vi "System_Read Module DVRs.vi"(11 "Data Value Reference in":refnum<data-value>) -> (2 "Dispatch Module DVR Array":refnum<data-value>[](array[refnum]), 3 "Data Value Reference out":refnum<data-value>)   [LabVIEW 2015, in "System.lvclass"]
uses:
  System.lvclass
  DispatchInterface/Interface_Dispatch.lvclass
  System.lvclass/System.ctl
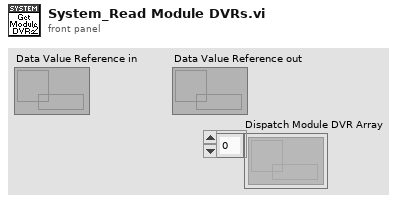
[diagram p1: front panel]
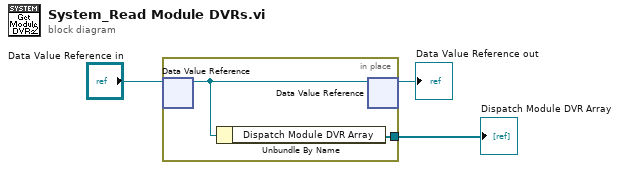
[diagram p0: block diagram]
diagram:
  n1 = in-place {
    in-place-border: [w4] -> w1
    n2 = in-place-dvr #1("Data Value Reference in") -> (w5:refnum<class "System.lvclass">)  [unwired: 1 out]
    n3 = Unbundle By Name(w5) -> ("Dispatch Module DVR Array"=w4:refnum<data-value>[])
    n4 = in-place-dvr #1(w5) -> (→"Data Value Reference out":refnum<data-value>)  [unwired: 1 out]
  }
  "Dispatch Module DVR Array" <- w1
